vi "BuildCmdText.vi"(3 "Command":string, 4 "ROS":T1, 5 "Name":enum16{"topic", "node"}(ring)) -> (2 "String":string)   [LabVIEW 2012]
uses:
  <userlib>/ROSforLV/ROS/Code/SubVIs/_ROSControl.ctl
  <userlib>/ROSforLV/ROS/Code/SubVIs/_ROSDirection.ctl
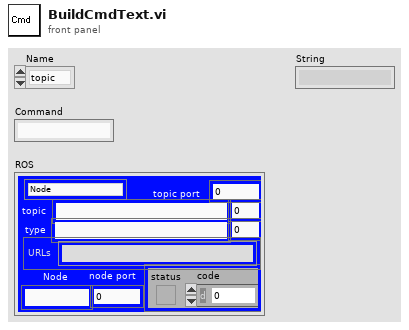
[diagram p1: front panel]
types:
  T1 = typedef "_ROSControl.ctl" = cluster{"topic port":u16, "Node":string, "topic":string, "type":string, "node port":u16, "error ":errorcluster, "Direction":T2, "APIs":string[], "Update (ms)":u16, "write queue":u16}
  T2 = typedef "_ROSDirection.ctl" = enum16{"Node", "Publisher", "Subscriber", "Service Client"}
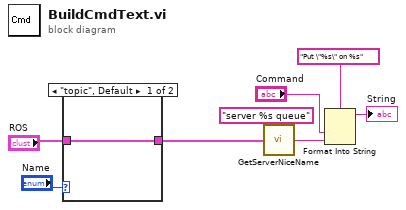
[diagram p0: block diagram]
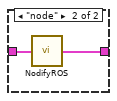
[diagram p2: hidden frame]
diagram:
  n1 = case shown="\"topic\", Default" "Name" {
    tunnel: "ROS" -> [w9 w11]
    tunnel: [w9 w10] -> w1
    frame "topic", Default {
    }
    frame "node" {
      n2 = call <userlib>:"NodifyROS.vi"("ROS in"=w11) -> ("ROS out"=w10:T1)
    }
  }
  n3 = call <userlib>:"GetServerNiceName.vi"("ROS"=w1, "Text to add"="server %s queue" ("format string")) -> ("String"=w3:string)
  n4 = Format Into String(format string="Put \"%s\" on %s", "Command", w3) -> (resulting string=→"String":string)  [unwired: 2 in, 1 out]
